vi "Interleaving1DArrays.vi"(10 "Unit":string[](array[string]), 11 "Property":string[](array[string])) -> (3 "Column Header":string)   [LabVIEW 2014]
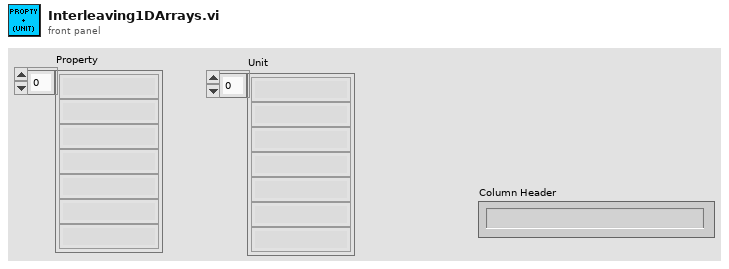
[diagram p1: front panel]
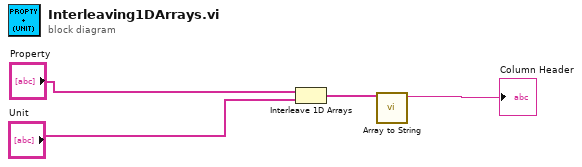
[diagram p0: block diagram]
diagram:
  n1 = Interleave 1D Arrays("Property", "Unit") -> (w1:string[])
  n2 = call "Array to String.vi"("Array"=w1) -> ("String"=→"Column Header":string)  [unwired: 10 in]
